vi "CONFIGURE PORTS.vi"() -> ()   [LabVIEW 2013]
uses:
  <vilib>/Instr/_visa.llb/VISA Configure Serial Port (Instr).vi
panel:
  out "LED":bool
  out "Current Address":string
  in  "stop":bool
  in  "Addresses":refnum<visa-resource-name>[](array[refnum])=["COM3", "COM4", "COM5", "COM6", "COM7", "COM8", "COM9", "COM10"]
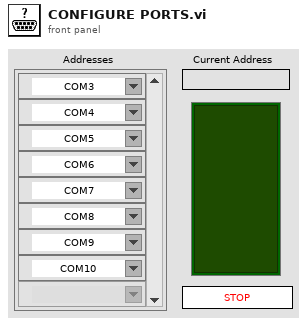
[diagram p1: front panel]
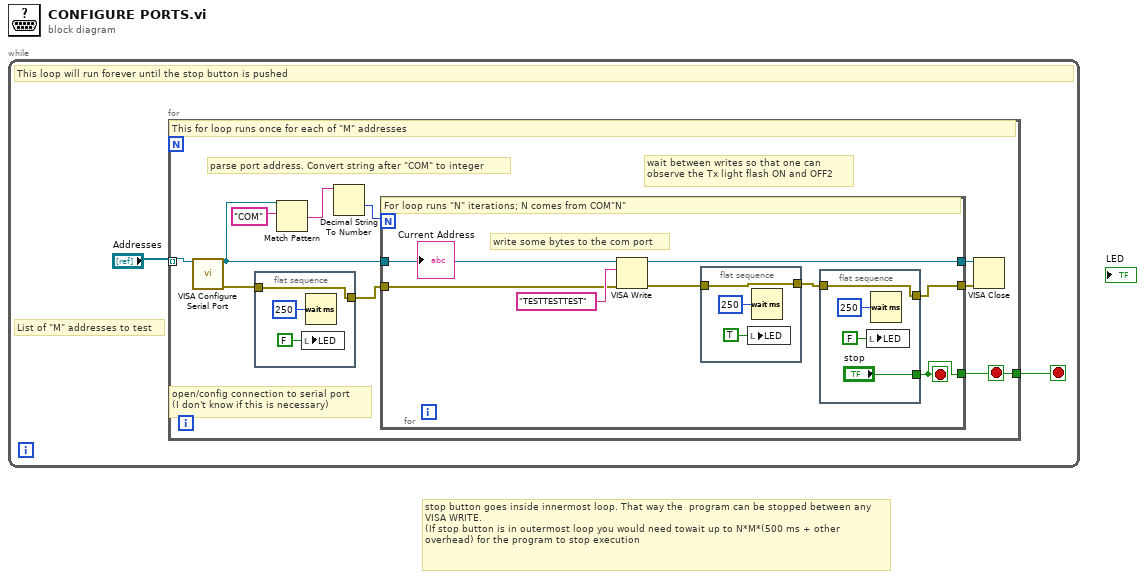
[diagram p0: block diagram]
diagram:
  # "stop button goes inside innermost loop. That way the  program can be stopped between any VISA WRITE.\n(If stop button is in outermost loop you would need towait up to N*M*(500 ms + other overhead) for the program to stop execution"
  n1 = while {
    stop <- w1 stop-if-true
    # "List of \"M\" addresses to test"
    # "This loop will run forever until the stop button is pushed"
    n2 = for {
      tunnel: "Addresses" -> [w12] mode=indexing
      tunnel: [w11] -> w1
      stop <- w11 stop-if-true
      # "wait between writes so that one can\nobserve the Tx light flash ON and OFF2"
      # "open/config connection to serial port\n(I don't know if this is necessary)"
      # "parse port address. Convert string after \"COM\" to integer"
      # "This for loop runs once for each of \"M\" addresses"
      n3 = call-poly "VISA Configure Serial Port"("VISA resource name"=w12) -> ("VISA resource name out"=w9:refnum<visa-resource-name>, "error out"=w4:errorcluster)  [unwired: 13 in]
      n4 = flat-sequence {
        tunnel: w4 -> [w13]
        tunnel: [w13] -> w3
        frame #0 {
          n5 = local write "LED"(FALSE ("LED")) -> ()
          n6 = Wait (ms)(milliseconds to wait=u32 250) -> ()  [unwired: 1 out]
        }
      }
      n7 = Match Pattern(string=w9, regular expression="COM") -> (after substring=w5:string)  [unwired: 1 in, 3 out]
      n8 = Decimal String To Number(string=w5) -> (number=w6:i32)  [unwired: 2 in, 1 out]
      n9 = for {
        N: w6 -> [_]
        tunnel: w9 -> [w21]
        tunnel: [w23] -> w7
        tunnel: w3 -> [w19]
        tunnel: [w17] -> w8
        tunnel: [w16] -> w11
        stop <- w16 stop-if-true
        # "write some bytes to the com port"
        # "For loop runs \"N\" iterations; N comes from COM\"N\""
        n10 = VISA Write(VISA resource name=w21, write buffer="TESTTESTTEST", error in (no error)=w19) -> (VISA resource name out=w23:refnum<visa-resource-name>, error out=w20:errorcluster)  [unwired: 1 out]
        n11 = flat-sequence {
          tunnel: w20 -> [w28]
          tunnel: [w28] -> w18
          frame #0 {
            n12 = local write "LED"(TRUE ("LED")) -> ()
            n13 = Wait (ms)(milliseconds to wait=u32 250) -> ()  [unwired: 1 out]
          }
        }
        n14 = flat-sequence {
          tunnel: w18 -> [w25]
          tunnel: [w25] -> w17
          tunnel: ["stop"] -> w16
          frame #0 {
            n15 = local write "LED"(FALSE ("LED")) -> ()
            n16 = Wait (ms)(milliseconds to wait=u32 250) -> ()  [unwired: 1 out]
          }
        }
        "Current Address" <- w21
      }
      n17 = VISA Close(VISA resource name=w7, error in (no error)=w8) -> ()  [unwired: 1 out]
    }
  }
